vi "Jenkins Unit Test.vi"(11 "Args":string[](array[string])) -> (2 "Output":string, 3 "Exit Code":i32)   [LabVIEW 2021]
uses:
  <vilib>/addons/_JKI Toolkits/Caraya/classes/Test Suite/Define Test Suite (JUnit Report).vi
  <vilib>/addons/_JKI Toolkits/Caraya/classes/Test Suite/Test Suite.lvclass
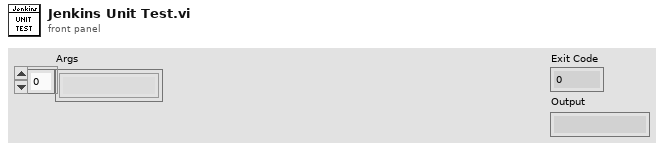
[diagram p1: front panel]
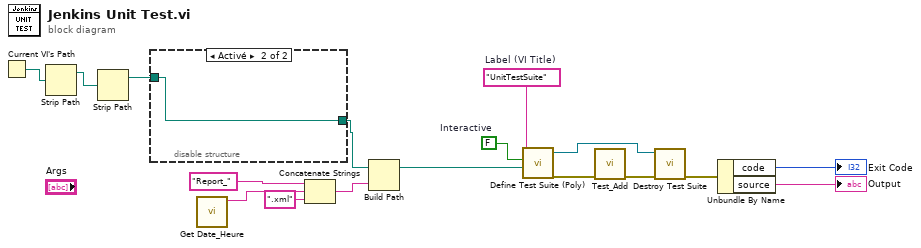
[diagram p0: block diagram]
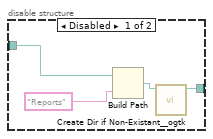
[diagram p2: hidden frame]
diagram:
  w16 = FALSE  # Interactive
  w17 = "UnitTestSuite"  # Label (VI Title)
  n1 = Current VI's Path() -> (path=w3:path)
  n2 = Strip Path(path=w3) -> (stripped path=w2:path)  [unwired: 1 out]
  n3 = Strip Path(path=w2) -> (stripped path=w1:path)  [unwired: 1 out]
  n4 = disable-structure shown="Activé" {
    disable-tunnel: [w19 w22] -> w13
    disable-tunnel: w1 -> [w18 w22]
    frame Disabled {
      n5 = Build Path(base path=w18, name or relative path="Reports") -> (appended path=w20:path)
      n6 = call <userlib>:"Create Dir if Non-Existant__ogtk.vi"("Directory Path"=w20) -> ("dup Directory Path"=w19:path)  [unwired: 8 in, 2 out]
    }
    frame Enabled {
    }
  }
  n7 = call "Get Date_Heure.vi"() -> ("Date_Heure"=w10:string)  [unwired: 11 in]
  n8 = Concatenate Strings("Report_" ("Report Path"), w10, ".xml" ("chaîne")) -> (w12:string)
  n9 = Build Path(base path=w13, name or relative path=w12) -> (appended path=w15:path)
  n10 = call-poly <vilib>:"Define Test Suite (Poly).vi"("Report Path"=w15, "Interactive"=w16, "Label (VI Title)"=w17) -> ("error out"=w9:errorcluster, "Test Suite"=w7:refnum<class "Test Suite.lvclass">)  [unwired: 6 in, 1 out]
  n11 = call "Test_Add.vi"("error in (no error)"=w9) -> ("error out"=w8:errorcluster)  [unwired: 10 in]
  n12 = call-dynamic "Destroy Test Suite.vi"("error in (no error)"=w8, "Test Suite in"=w7) -> ("error out"=w4:errorcluster)  [unwired: 8 in, 1 out]
  n13 = Unbundle By Name(w4) -> ("code"=→"Exit Code":i32, "source"=→"Output":string)
